vi "Close Nested.vi"(8 "error in (no error)":errorcluster, 10 "Nested":T1, 11 "Open Close Logic Simple Table in":refnum<class "Open Close Logic Simple Table.lvclass">) -> (0 "error out":errorcluster, 3 "Open Close Logic Simple Table out":refnum<class "Open Close Logic Simple Table.lvclass">)   [LabVIEW 2020, in "Open Close Logic Simple Table.lvlib" / "Open Close Logic Simple Table.lvclass"]
uses:
  Open Close Logic Simple Table.lvclass
  Form ID.ctl
  Open Close Logic Simple Table.lvclass/Open Close Logic Simple Table.ctl
  <userlib>/_OpenG.lib/array/array.llb/Search 1D Array (Variant)__ogtk.vi
  <userlib>/_OpenG.lib/array/array.llb/Delete Elements from 1D Array (Variant)__ogtk.vi
  Form Server Interfaces.lvlib
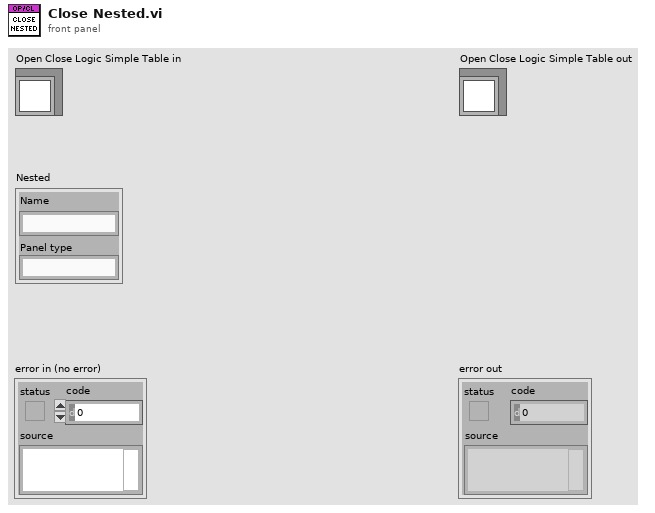
[diagram p1: front panel]
types:
  T1 = typedef "Form Server Interfaces.lvlib/Form ID.ctl" = cluster{"Name":string, "Panel type":string}
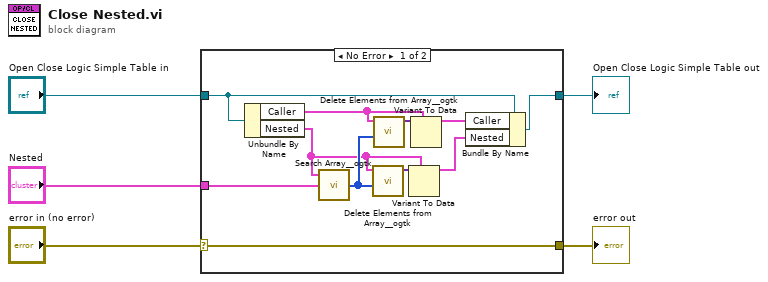
[diagram p0: block diagram]
diagram:
  n1 = case shown="No Error" "error in (no error)" {
    selector: "error in (no error)" -> [w16 w18]
    tunnel: [w16 w18] -> w4
    tunnel: "Open Close Logic Simple Table in" -> [w9 w17]
    tunnel: [w6 w17] -> w2
    tunnel: "Nested" -> [w15 _]
    frame No Error {
      n2 = Unbundle By Name(w9) -> ("Caller"=w12:T1[], "Nested"=w10:T1[])
      n3 = call-poly <userlib>:"Search Array__ogtk.vi"("Array"=w10, "Element Data"=w15) -> ("Indices of Elements"=w14:i32[])  [unwired: 7 in]
      n4 = call-poly <userlib>:"Delete Elements from Array__ogtk.vi"("indices"=w14, "array"=w10) -> ("array w/ subset deleted"=w11:variant[])  [unwired: 8 in, 1 out]
      n5 = call-poly <userlib>:"Delete Elements from Array__ogtk.vi"("indices"=w14, "array"=w12) -> ("array w/ subset deleted"=w13:variant[])  [unwired: 8 in, 1 out]
      n6 = Variant To Data(type=w10, Variant=w11) -> (data=w7:T1[])  [unwired: 1 in, 1 out]
      n7 = Variant To Data(type=w12, Variant=w13) -> (data=w8:T1[])  [unwired: 1 in, 1 out]
      n8 = Bundle By Name(cluster=w9, "Caller"=w8, "Nested"=w7) -> (w6:refnum<class "Open Close Logic Simple Table.lvclass">)
    }
    frame Error {
    }
  }
  "error out" <- w4
  "Open Close Logic Simple Table out" <- w2
